vi "sequence structure.vi"() -> ()   [LabVIEW 2020]
panel:
  out "Numeric 3":dbl format="%#_13g"
  out "x/y":dbl
  out "x-y":dbl
  out "x+y":dbl
  in  "Numeric 2":dbl format="%#_13g"
  in  "Numeric":dbl format="%#_13g"
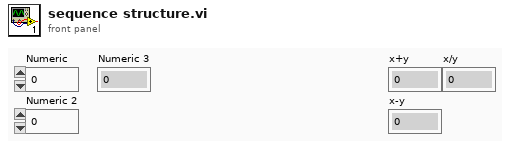
[diagram p1: front panel]
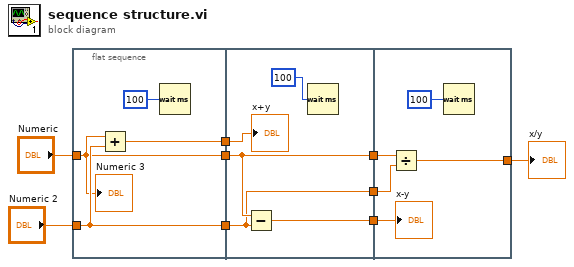
[diagram p0: block diagram]
diagram:
  n1 = flat-sequence {
    tunnel: [w10] -> w9
    tunnel: "Numeric" -> [w10]
    tunnel: [w13] -> w6
    tunnel: "Numeric 2" -> [w13]
    tunnel: [w12] -> w1
    tunnel: w9 -> [w18]
    tunnel: [w18] -> w7
    tunnel: w6 -> [w17]
    tunnel: [w17] -> w4
    tunnel: [w16] -> w2
    tunnel: w1 -> [w15]
    tunnel: w7 -> [w23]
    tunnel: w4 -> [w22]
    tunnel: [w21] -> w3
    tunnel: w2 -> [w20]
    frame #0 {
      n2 = Add(x=w10, y=w13) -> (x+y=w12:dbl)
      n3 = Wait (ms)(milliseconds to wait=u32 100) -> ()  [unwired: 1 out]
      "Numeric 3" <- w10
    }
    frame #1 {
      n4 = Subtract(x=w18, y=w17) -> (x-y=w16:dbl)
      n5 = Wait (ms)(milliseconds to wait=u32 100) -> ()  [unwired: 1 out]
      "x+y" <- w15
    }
    frame #2 {
      n6 = Divide(x=w23, y=w22) -> (x/y=w21:dbl)
      n7 = Wait (ms)(milliseconds to wait=u32 100) -> ()  [unwired: 1 out]
      "x-y" <- w20
    }
  }
  "x/y" <- w3
